vi "Write_Waveform.vi"(8 "Error_In":errorcluster, 10 "I2C_Waveform":waveform(dbl)[](graph), 11 "I2C_In":refnum<class "I2C.lvclass">) -> (0 "Error_Out":errorcluster, 3 "I2C_Out":refnum<class "I2C.lvclass">)   [LabVIEW 2023, in "I2C.lvclass"]
doc: "Used to Write the I2C Waveform"
uses:
  I2C.lvclass
  I2C.lvclass/I2C.ctl
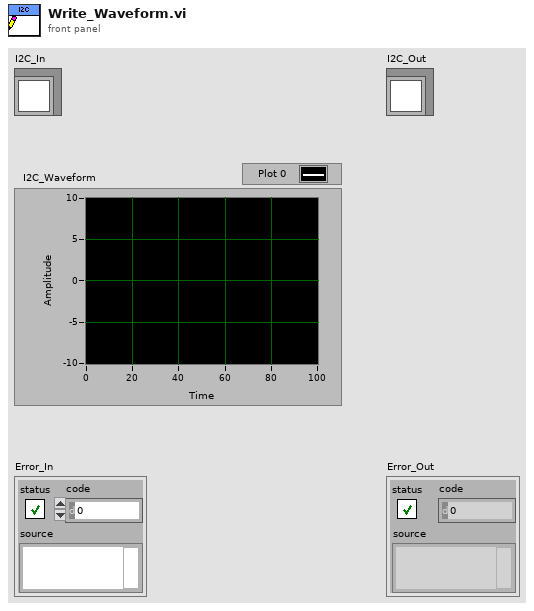
[diagram p1: front panel]
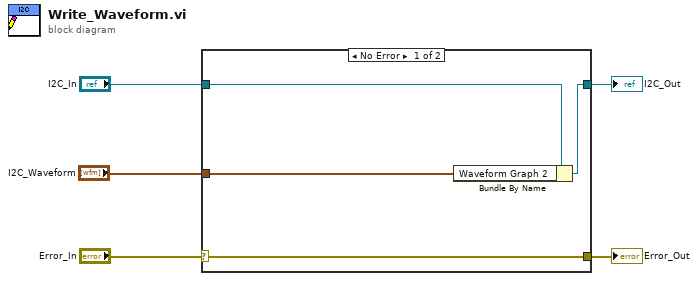
[diagram p0: block diagram]
diagram:
  n1 = case shown="No Error" "Error_In" {
    selector: "Error_In" -> [w9 w10]
    tunnel: [w9 w10] -> w4
    tunnel: [w7 w11] -> w2
    tunnel: "I2C_In" -> [w8 w11]
    tunnel: "I2C_Waveform" -> [w6 _]
    frame No Error {
      n2 = Bundle By Name(cluster=w8, "Waveform Graph 2"=w6) -> (w7:refnum<class "I2C.lvclass">)
    }
    frame Error {
    }
  }
  "Error_Out" <- w4
  "I2C_Out" <- w2
